vi "Parse_Sound.vi"(8 "error in (no error)":errorcluster, 11 "JSON String":string) -> (0 "error out":errorcluster, 1 "Found?":bool, 2 "Sound File Name":string, 3 "JSON String Out":string)   [LabVIEW 2018, in "MerriamWebsterJSON.lvlib"]
uses:
  MerriamWebsterJSON.lvlib
  <vilib>/LVH/i3 JSON/JSON Parsing/Get Array Value at Index Files/Get Array Value at Index - Object.vi
  <vilib>/LVH/i3 JSON/JSON Parsing/Get Object Parameter Files/Get Object Parameter - Object.vi
  <vilib>/LVH/i3 JSON/JSON Parsing/Get Object Parameter Files/Get Object Parameter - String.vi
  <vilib>/LVH/i3 JSON/i3-json.lvlib
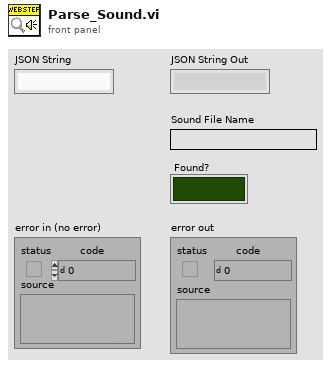
[diagram p1: front panel]
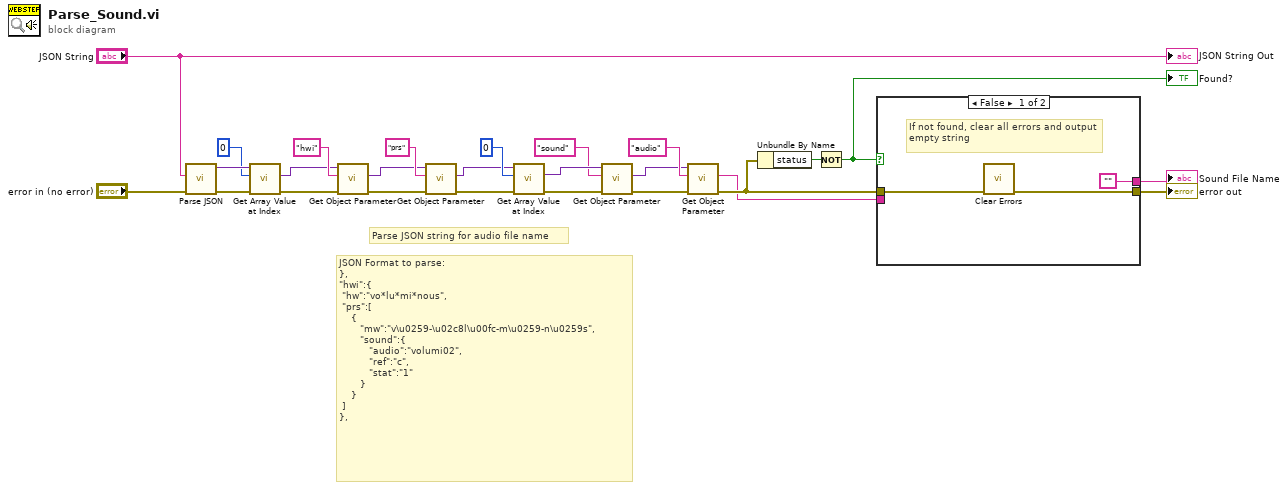
[diagram p0: block diagram]
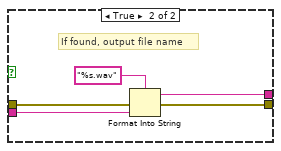
[diagram p2: hidden frame]
diagram:
  # "JSON Format to parse:\n},\n\"hwi\":{  \n \"hw\":\"vo*lu*mi*nous\",\n \"prs\":[  \n    {  \n       \"mw\":\"v\\u0259-\\u02c8l\\u00fc-m\\u0259-n\\u0259s\",\n       \"sound\":{  \n          \"audio\":\"volumi02\",\n          \"ref\":\"c\",\n          \"stat\":\"1\"\n       }\n    }\n ]\n},"
  # "Parse JSON string for audio file name"
  n1 = call <vilib>:"Parse JSON.vi"("error in (no error)"="error in (no error)", "JSON String"="JSON String") -> ("error out"=w20:errorcluster, "JSON Tree"=w26:variant)  [unwired: 6 in, 2 out]
  n2 = call-poly <vilib>:"Get Array Value at Index.vi"("error in (no error)"=w20, "Index"=0, "JSON Tree In (JSON Array)"=w26) -> ("error out"=w21:errorcluster, "JSON Object"=w23:variant)  [unwired: 5 in, 2 out]
  n3 = call-poly <vilib>:"Get Object Parameter.vi"("error in (no error)"=w21, "Parameter Name"="hwi", "JSON Tree In (JSON Object)"=w23) -> ("error out"=w5:errorcluster, "JSON Object"=w6:variant)  [unwired: 5 in, 2 out]
  n4 = call-poly <vilib>:"Get Object Parameter.vi"("error in (no error)"=w5, "Parameter Name"="prs", "JSON Tree In (JSON Object)"=w6) -> ("error out"=w9:errorcluster, "JSON Object"=w10:variant)  [unwired: 5 in, 2 out]
  n5 = call-poly <vilib>:"Get Array Value at Index.vi"("error in (no error)"=w9, "Index"=0, "JSON Tree In (JSON Array)"=w10) -> ("error out"=w8:errorcluster, "JSON Object"=w15:variant)  [unwired: 5 in, 2 out]
  n6 = call-poly <vilib>:"Get Object Parameter.vi"("error in (no error)"=w8, "Parameter Name"="sound", "JSON Tree In (JSON Object)"=w15) -> ("error out"=w7:errorcluster, "JSON Object"=w12:variant)  [unwired: 5 in, 2 out]
  n7 = call-poly <vilib>:"Get Object Parameter.vi"("error in (no error)"=w7, "Parameter Name"="audio", "JSON Tree In (JSON Object)"=w12) -> ("error out"=w4:errorcluster, "String Value"=w2:string)  [unwired: 5 in, 2 out]
  n8 = Unbundle By Name(w4) -> ("status"=w18:bool)
  n9 = Not(x=w18) -> (.not. x?=w17:bool)
  "Found?" <- w17
  n10 = case shown="False" w17 {
    tunnel: w4 -> [w29 w34]
    tunnel: [w28 w33] -> w3
    tunnel: w2 -> [_ w30]
    tunnel: ["" w31] -> w1
    frame False {
      # "If not found, clear all errors and output empty string"
      n11 = call <vilib>:"Clear Errors.vi"("error in (no error)"=w29) -> ("error out"=w28:errorcluster)  [unwired: 5 in, 1 out]
    }
    frame True {
      # "If found, output file name"
      n12 = Format Into String(format string="%s.wav", error in=w34, w30) -> (resulting string=w31:string, error out=w33:errorcluster)  [unwired: 1 in]
    }
  }
  "error out" <- w3
  "Sound File Name" <- w1
  "JSON String Out" <- "JSON String"
